vi "Random range (SubVI).vi"(11 "Ranges":dbl[](array[numeric])) -> (1 "Rondom value":dbl, 3 "Index":i32)   [LabVIEW 2013]
doc: "Generates an element and assign its range to the input ranges. \n\nE.g. input ranges are 5, 1, 2 then there is 1/8 of chance the generated value is in the 2nd range.\nNote: the input ranges must be positive values."
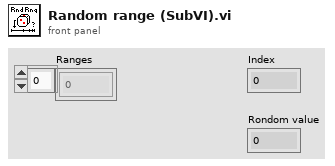
[diagram p1: front panel]
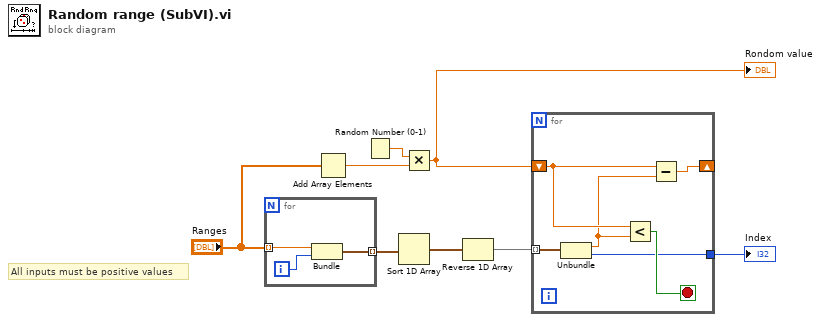
[diagram p0: block diagram]
diagram:
  # "All inputs must be positive values"
  n1 = for {
    tunnel: "Ranges" -> [w11] mode=indexing
    tunnel: [w9] -> w7 mode=indexing
    i -> [w10]
    n2 = Bundle("element"=w11, w10) -> (w9:cluster{"element":dbl, i32})  [unwired: 1 in]
  }
  n3 = Add Array Elements(numeric array="Ranges") -> (sum=w4:dbl)
  n4 = Random Number (0-1)() -> (number: 0 to 1=w3:dbl)
  n5 = Sort 1D Array(array=w7) -> (sorted array=w6:cluster{"element":dbl, i32}[])
  n6 = Multiply(x=w3, y=w4) -> (x*y=w1:dbl)
  "Rondom value" <- w1
  n7 = Reverse 1D Array(array=w6) -> (reversed array=w2:cluster{"element":dbl, i32}[])
  n8 = for {
    tunnel: w2 -> [w17] mode=indexing
    shift-right: [w14] -> _
    shift-left: w1 -> [w16]
    tunnel: [w12] -> w8
    stop <- w13 stop-if-true
    n9 = Unbundle(w17) -> ("element"=w15:dbl, w12:i32)
    n10 = Less?(x=w16, y=w15) -> (x < y?=w13:bool)
    n11 = Subtract(x=w16, y=w15) -> (x-y=w14:dbl)
  }
  "Index" <- w8
